vi "4.4.vi"() -> ()   [LabVIEW 2017]
panel:
  in  "温度":dbl
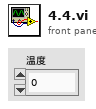
[diagram p1: front panel]
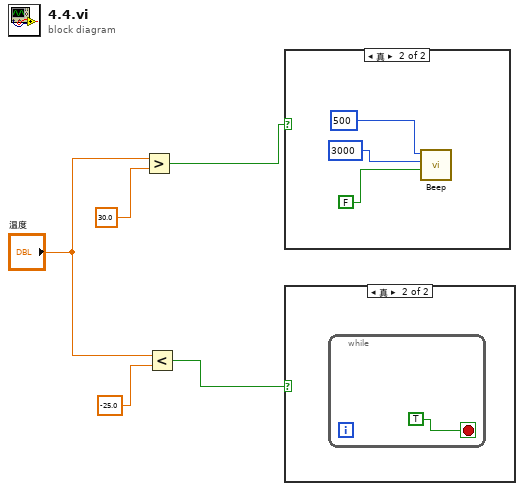
[diagram p0: block diagram]
diagram:
  n1 = Greater?(x="温度", y=30.0) -> (0:w4:bool)
  n2 = Less?(x="温度", y=-25.0) -> (x < y?=w1:bool)
  n3 = case shown="真" w4 {
    frame False {
    }
    frame True {
      n4 = call <vilib>:"Beep.vi"("use system alert? (T)"=FALSE, "duration (msec)"=3000, "frequency (Hz)"=500) -> ()  [unwired: 9 in]
    }
  }
  n5 = case shown="真" w1 {
    frame False {
    }
    frame True {
      n6 = while {
        stop <- TRUE stop-if-true
      }
    }
  }
